vi "Enqueue User Que (Normal).vi"(6 "モード(Normal)":enum16{"Normal", "Lossy", "OppositeEnd"}(ring), 7 "コマンド":string, 8 "エラー入力（エラーなし）":errorcluster, 9 "タイムアウト（ms）（-1）":i32=-1, 10 "バリアント":variant, 11 "queVariant":refnum<queue>) -> (0 "エラー出力":errorcluster, 1 "timeout/overflow?":bool, 3 "queVariant(copy)":refnum<queue>)   [LabVIEW 2016]
uses:
  Event/Ctl/EventVariantData.ctl
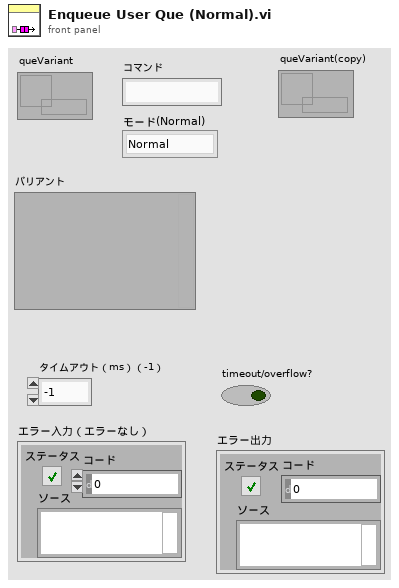
[diagram p1: front panel]
types:
  T1 = typedef "EventVariantData.ctl" = cluster{"コマンド":string, "バリアント":variant}
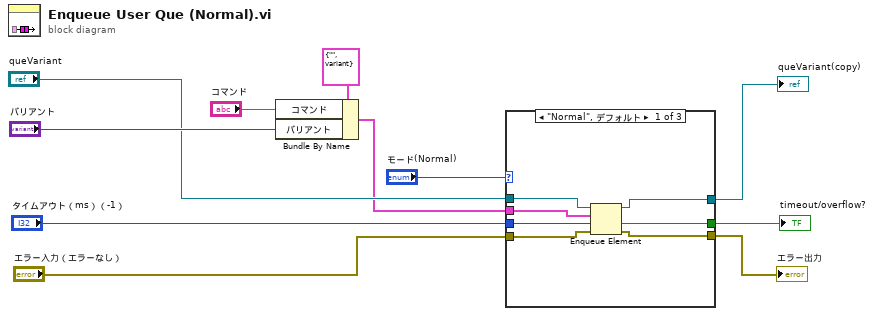
[diagram p0: block diagram]
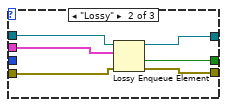
[diagram p2: hidden frame]
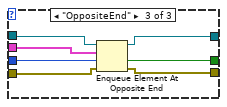
[diagram p3: hidden frame]
diagram:
  n1 = Bundle By Name(cluster=T1 {"コマンド"="", "バリアント"=variant} ("要素"), "コマンド"="コマンド", "バリアント"="バリアント") -> (w5:T1)
  n2 = case shown="\"Normal\", デフォルト" "モード(Normal)" {
    tunnel: [w13 w24 w26] -> w11
    tunnel: "タイムアウト（ms）（-1）" -> [w17 _ w29]
    tunnel: "queVariant" -> [w18 w23 w31]
    tunnel: [w12 w22 w25] -> w7
    tunnel: w5 -> [w16 w21 w30]
    tunnel: "エラー入力（エラーなし）" -> [w15 w19 w28]
    tunnel: [w14 w20 w27] -> w2
    frame "Normal", Default {
      n3 = Enqueue Element(queue=w18, element=w16, timeout in ms (-1)=w17, error in (no error)=w15) -> (queue out=w12:refnum<queue>, timed out?=w13:bool, error out=w14:errorcluster)
    }
    frame "Lossy" {
      n4 = Lossy Enqueue Element(queue=w23, element=w21, error in (no error)=w19) -> (queue out=w22:refnum<queue>, overflow?=w24:bool, error out=w20:errorcluster)  [unwired: 1 out]
    }
    frame "OppositeEnd" {
      n5 = Enqueue Element At Opposite End(queue=w31, element=w30, timeout in ms (-1)=w29, error in (no error)=w28) -> (queue out=w25:refnum<queue>, timed out?=w26:bool, error out=w27:errorcluster)
    }
  }
  "timeout/overflow?" <- w11
  "エラー出力" <- w2
  "queVariant(copy)" <- w7
